vi "relayShortCircuitTest.vi"() -> ()   [LabVIEW 2023]
panel:
  in  "CV":bool
  in  "relay 2 (unshort)":bool
  in  "switchTime/s":i32=50
  in  "flag 2":bool
  out "error out":errorcluster
  in  "error in (no error)":errorcluster
  in  "VISA relay":refnum<visa-resource-name>
  in  "VISA 2110 current":refnum<visa-resource-name>="USB0::0x05E6::0x2110::8017058::INSTR"
  in  "VISA 2110 voltage":refnum<visa-resource-name>="USB0::0x05E6::0x2110::8016020::INSTR"
  out "error out 4":errorcluster
  out "error out 3":errorcluster
  in  "stop 5":bool
  out "Current through 330 ohm resistor inner segment/mA 6":cluster{"Y":dbl[], "Y":dbl[]}[](graph)
  out "Voltage across 330 ohm resistor 7":dbl[](graph)
  out "Voltage across 330 ohm resistor 8":dbl[](array[numeric])
  out "Current time":timestamp
  out "Voltage/V":cluster{"Y":dbl[], "Y":dbl[]}[](graph)
  out "Voltage":dbl[](graph)
  out "Voltage":dbl[](array[numeric])
  in  "Filename 4":path caption="Filename"
  in  "Camera":bool
  out "Start time":timestamp
  in  "Countdown/s":i32=3
  out "Timer":dbl
  in  "error in (no error) 3":errorcluster
  in  "error in (no error) 2":errorcluster
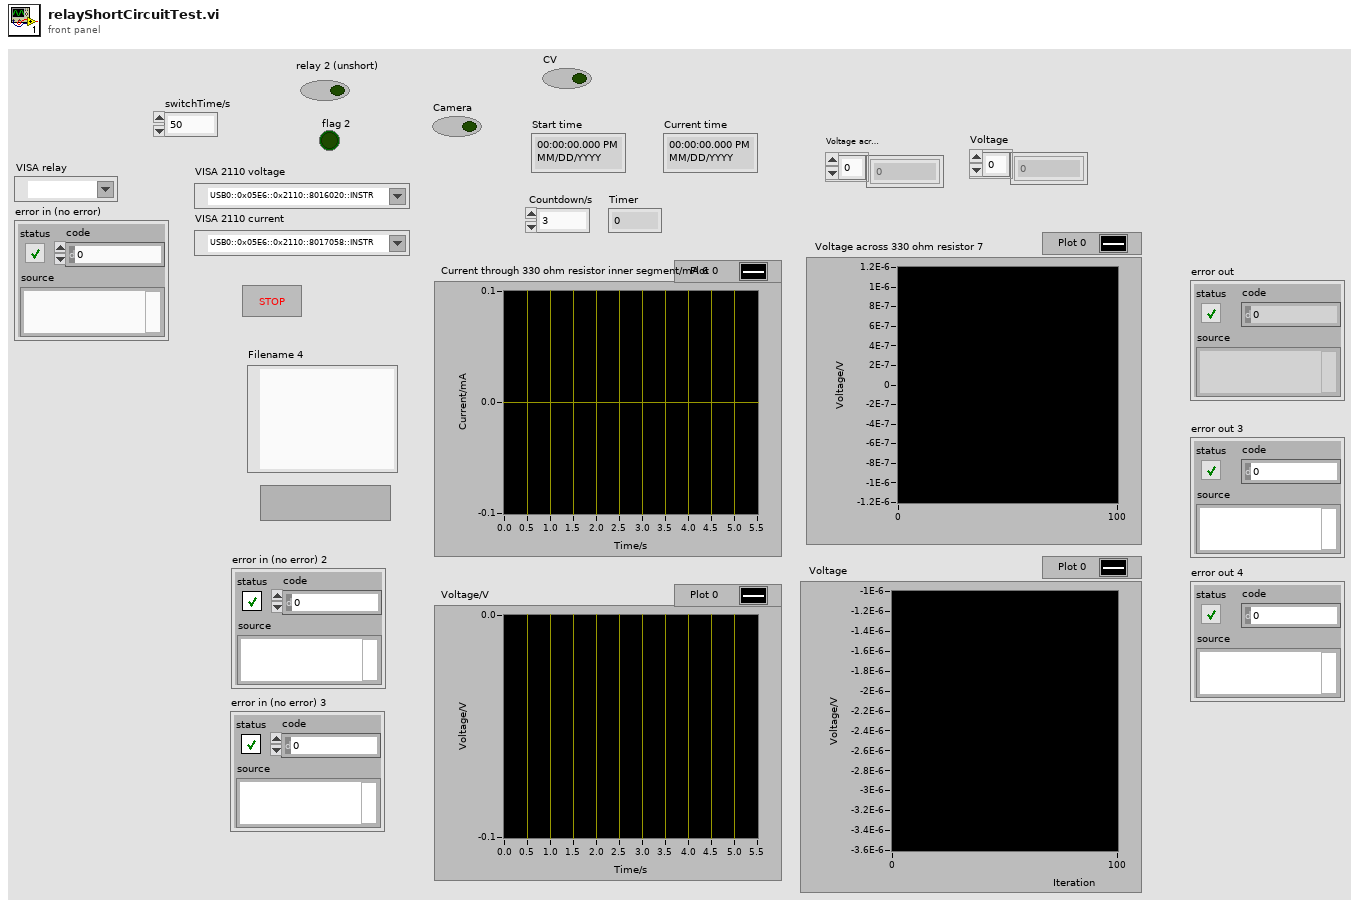
[diagram p1: front panel]
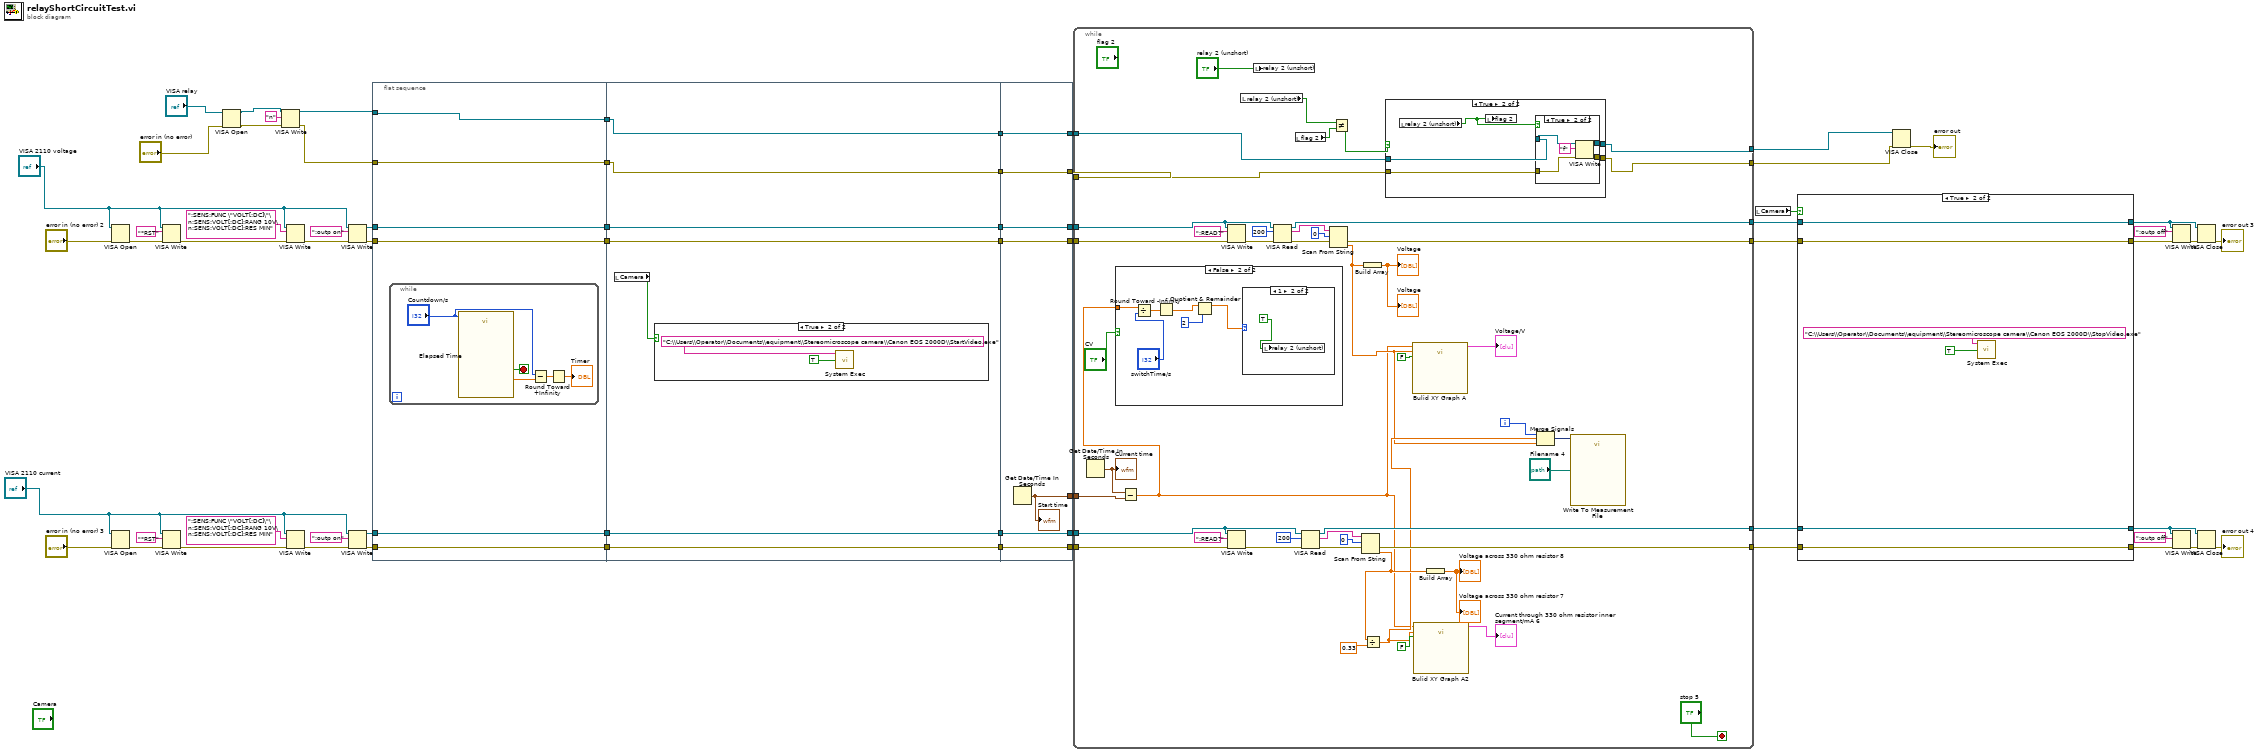
[diagram p0: block diagram]
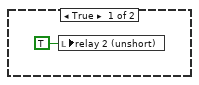
[diagram p3: hidden frame]
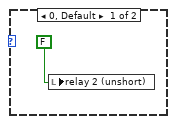
[diagram p4: hidden frame]
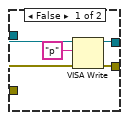
[diagram p6: hidden frame]
diagram:
  n1 = VISA Open(error in (no error)="error in (no error) 2", VISA resource name="VISA 2110 voltage") -> (error out=w64:errorcluster)  [unwired: 3 in, 1 out]
  n2 = VISA Open(error in (no error)="error in (no error) 3", VISA resource name="VISA 2110 current") -> (error out=w58:errorcluster)  [unwired: 3 in, 1 out]
  n3 = VISA Write(VISA resource name="VISA 2110 voltage", write buffer="*RST" ("数据"), error in (no error)=w64) -> (error out=w63:errorcluster)  [unwired: 2 out]
  n4 = VISA Write(VISA resource name="VISA 2110 current", write buffer="*RST" ("数据"), error in (no error)=w58) -> (error out=w57:errorcluster)  [unwired: 2 out]
  n5 = VISA Open(error in (no error)="error in (no error)", VISA resource name="VISA relay") -> (VISA resource name=w4:refnum<visa-resource-name>, error out=w3:errorcluster)  [unwired: 3 in]
  n6 = VISA Write(VISA resource name=w4, write buffer="n", error in (no error)=w3) -> (VISA resource name out=w1:refnum<visa-resource-name>, error out=w2:errorcluster)  [unwired: 1 out]
  n7 = VISA Write(VISA resource name="VISA 2110 voltage", write buffer=":SENS:FUNC \"VOLT[:DC]\"\n:SENS:VOLT[:DC]:RANG 10V\n:SENS:VOLT[:DC]:RES MIN" ("address string"), error in (no error)=w63) -> (error out=w62:errorcluster)  [unwired: 2 out]
  n8 = VISA Write(VISA resource name="VISA 2110 current", write buffer=":SENS:FUNC \"VOLT[:DC]\"\n:SENS:VOLT[:DC]:RANG 10V\n:SENS:VOLT[:DC]:RES MIN" ("address string"), error in (no error)=w57) -> (error out=w56:errorcluster)  [unwired: 2 out]
  n9 = VISA Write(VISA resource name="VISA 2110 voltage", write buffer=":outp on" ("数据"), error in (no error)=w62) -> (VISA resource name out=w42:refnum<visa-resource-name>, error out=w41:errorcluster)  [unwired: 1 out]
  n10 = VISA Write(VISA resource name="VISA 2110 current", write buffer=":outp on" ("数据"), error in (no error)=w56) -> (VISA resource name out=w40:refnum<visa-resource-name>, error out=w39:errorcluster)  [unwired: 1 out]
  n11 = flat-sequence {
    tunnel: w41 -> [w69]
    tunnel: w42 -> [w70]
    tunnel: [w70] -> w50
    tunnel: [w69] -> w49
    tunnel: w40 -> [w68]
    tunnel: [w68] -> w48
    tunnel: w39 -> [w67]
    tunnel: [w67] -> w47
    tunnel: [w66] -> w14
    tunnel: w1 -> [w66]
    tunnel: [w65] -> w11
    tunnel: w2 -> [w65]
    tunnel: w50 -> [w82]
    tunnel: w49 -> [w81]
    tunnel: [w82] -> w46
    tunnel: [w81] -> w45
    tunnel: [w79] -> w44
    tunnel: w48 -> [w79]
    tunnel: [w78] -> w43
    tunnel: w47 -> [w78]
    tunnel: w14 -> [w77]
    tunnel: [w77] -> w13
    tunnel: w11 -> [w76]
    tunnel: [w76] -> w10
    tunnel: [w89] -> w38
    tunnel: [w90] -> w36
    tunnel: [w91] -> w37
    tunnel: w46 -> [w91]
    tunnel: w45 -> [w90]
    tunnel: [w88] -> w35
    tunnel: w44 -> [w88]
    tunnel: [w87] -> w34
    tunnel: w43 -> [w87]
    tunnel: [w86] -> w12
    tunnel: w13 -> [w86]
    tunnel: [w85] -> w9
    tunnel: w10 -> [w85]
    frame #0 {
      n12 = while {
        stop <- w73 stop-if-true
        n13 = call "Elapsed Time"("Time Target (s)"="Countdown/s") -> ("Elapsed Time (s)"=w75:dbl, "Time has Elapsed"=w73:bool)  [unwired: 11 in, 6 out]
        n14 = Subtract(x="Countdown/s", y=w75) -> (x-y=w72:dbl)
        n15 = Round Toward +Infinity(x=w72) -> (ceil(x): smallest int >= x=→"Timer":dbl)
      }
    }
    frame #1 {
      n16 = local read "Camera"() -> (w80:bool)
      n17 = case shown="True" w80 {
        frame False {
        }
        frame True {
          n18 = call <vilib>:"System Exec.vi"("wait until completion? (T)"=TRUE, "command line"="C:\\Users\\Operator\\Documents\\equipment\\Stereomicroscope camera\\Canon EOS 2000D\\StartVideo.exe") -> ()  [unwired: 6 in, 4 out]
        }
      }
    }
    frame #2 {
      n19 = Get Date/Time In Seconds() -> (seconds since 1Jan1904=w89:timestamp)
      "Start time" <- w89
    }
  }
  n20 = while {
    tunnel: w38 -> [w137]
    tunnel: w37 -> [w136]
    tunnel: w36 -> [w135]
    tunnel: w35 -> [w134]
    tunnel: w34 -> [w133]
    tunnel: [w131] -> w26
    tunnel: [w130] -> w24
    tunnel: [w129] -> w22
    tunnel: [w128] -> w20
    tunnel: w12 -> [w123]
    tunnel: w9 -> [w124]
    tunnel: [w97] -> w8
    tunnel: [w96] -> w7
    i -> [w127]
    stop <- "stop 5" stop-if-true
    n21 = Get Date/Time In Seconds() -> (seconds since 1Jan1904=w105:timestamp)
    "Current time" <- w105
    n22 = Subtract(x=w105, y=w137) -> (x-y=w95:dbl)
    n23 = case shown="False" "CV" {
      tunnel: w95 -> [_ w141]
      frame True {
        n24 = local write "relay 2 (unshort)"(TRUE ("relay 2 (unshort)")) -> ()
      }
      frame False {
        n25 = Divide(x=w141, y="switchTime/s") -> (x/y=w144:dbl)
        n26 = Round Toward -Infinity(1:w144) -> (0:w143:dbl)
        n27 = Quotient & Remainder(x=w143, y=2) -> (x-y*floor(x/y)=w139:dbl)  [unwired: 1 out]
        n28 = case shown="1" w139 {
          frame 0, Default {
            n29 = local write "relay 2 (unshort)"(FALSE) -> ()
          }
          frame 1 {
            n30 = local write "relay 2 (unshort)"(TRUE) -> ()
          }
        }
      }
    }
    n31 = VISA Write(VISA resource name=w136, write buffer=":READ?" ("数据"), error in (no error)=w135) -> (error out=w118:errorcluster)  [unwired: 2 out]
    n32 = VISA Write(VISA resource name=w134, write buffer=":READ?" ("数据"), error in (no error)=w133) -> (error out=w109:errorcluster)  [unwired: 2 out]
    n33 = local read "relay 2 (unshort)"() -> (w93:bool)
    n34 = local write "relay 2 (unshort)"("relay 2 (unshort)") -> ()
    n35 = VISA Read(VISA resource name=w136, byte count=200 ("字节总数"), error in (no error)=w118) -> (VISA resource name out=w131:refnum<visa-resource-name>, read buffer=w120:string, error out=w119:errorcluster)  [unwired: 1 out]
    n36 = local read "flag 2"() -> (w126:bool)
    n37 = VISA Read(VISA resource name=w134, byte count=200 ("字节总数"), error in (no error)=w109) -> (VISA resource name out=w129:refnum<visa-resource-name>, read buffer=w111:string, error out=w110:errorcluster)  [unwired: 1 out]
    n38 = Scan From String(input string=w120, initial scan location=u32 0 ("初始扫描位置"), error in=w119) -> (error out=w130:errorcluster, output 1=w98:dbl)  [unwired: 2 in, 2 out]
    n39 = Not Equal?(x=w93, y=w126) -> (x != y?=w125:bool)
    n40 = Scan From String(input string=w111, initial scan location=u32 0 ("初始扫描位置"), error in=w110) -> (error out=w128:errorcluster, output 1=w100:dbl)  [unwired: 2 in, 2 out]
    n41 = Build Array(w98) -> (→"Voltage" →"Voltage":dbl[])
    n42 = Divide(x=w100, y=0.33) -> (x/y=w99:dbl)
    n43 = case shown="True" w125 {
      tunnel: w124 -> [w148 w150]
      tunnel: [w147 w153] -> w97
      tunnel: [w148 w152] -> w96
      tunnel: w123 -> [w147 w151]
      frame False {
      }
      frame True {
        n44 = local read "relay 2 (unshort)"() -> (w149:bool)
        n45 = local write "flag 2"(w149) -> ()
        n46 = case shown="True" w149 {
          tunnel: w151 -> [w155 w163]
          tunnel: w150 -> [w154 w161]
          tunnel: [w157 w160] -> w153
          tunnel: [w156 w159] -> w152
          frame False {
            n47 = VISA Write(VISA resource name=w155, write buffer="p", error in (no error)=w154) -> (VISA resource name out=w157:refnum<visa-resource-name>, error out=w156:errorcluster)  [unwired: 1 out]
          }
          frame True {
            n48 = VISA Write(VISA resource name=w163, write buffer="f", error in (no error)=w161) -> (VISA resource name out=w160:refnum<visa-resource-name>, error out=w159:errorcluster)  [unwired: 1 out]
          }
        }
      }
    }
    n49 = call "Bulid XY Graph A"("Reset"=FALSE, "Y Input"=w98, "X Input"=w95) -> ("XY Graph"=→"Voltage/V":cluster{"X":dbl[], "Y":dbl[]}[])  [unwired: 7 in, 1 out]
    n50 = call "Bulid XY Graph A2"("Reset"=FALSE, "Y Input"=w99, "X Input"=w95) -> ("XY Graph"=→"Current through 330 ohm resistor inner segment/mA 6":cluster{"X":dbl[], "Y":dbl[]}[])  [unwired: 7 in, 1 out]
    n51 = Build Array(w100) -> (→"Voltage across 330 ohm resistor 8" →"Voltage across 330 ohm resistor 7":dbl[])
    n52 = Merge Signals(w127, w99, w98) -> (w122:dynamicdata)
    n53 = call "Write To Measurement File"("Signals"=w122, "Filename"="Filename 4") -> ()  [unwired: 15 in, 3 out]
  }
  n54 = local read "Camera"() -> (w27:bool)
  n55 = case shown="True" w27 {
    tunnel: [w167 w171] -> w25
    tunnel: w26 -> [w167 w171]
    tunnel: [w166 w170] -> w23
    tunnel: w24 -> [w166 w170]
    tunnel: [w165 w169] -> w21
    tunnel: w22 -> [w165 w169]
    tunnel: [w164 w168] -> w19
    tunnel: w20 -> [w164 w168]
    frame False {
    }
    frame True {
      n56 = call <vilib>:"System Exec.vi"("wait until completion? (T)"=TRUE, "command line"="C:\\Users\\Operator\\Documents\\equipment\\Stereomicroscope camera\\Canon EOS 2000D\\StopVideo.exe") -> ()  [unwired: 6 in, 4 out]
    }
  }
  n57 = VISA Close(VISA resource name=w8, error in (no error)=w7) -> (error out=→"error out":errorcluster)
  n58 = VISA Write(VISA resource name=w25, write buffer=":outp off" ("数据"), error in (no error)=w23) -> (error out=w32:errorcluster)  [unwired: 2 out]
  n59 = VISA Write(VISA resource name=w21, write buffer=":outp off" ("数据"), error in (no error)=w19) -> (error out=w29:errorcluster)  [unwired: 2 out]
  n60 = VISA Close(VISA resource name=w25, error in (no error)=w32) -> (error out=→"error out 3":errorcluster)
  n61 = VISA Close(VISA resource name=w21, error in (no error)=w29) -> (error out=→"error out 4":errorcluster)
